vi "FGV Protokoll.vi"(6 "Enum":T1, 8 "error in (no error)":errorcluster caption="Fehler (Eingang, kein Fehler)", 9 "Graph2":waveform(dbl)[](graph), 10 "Pfad":path, 11 "Boolesch":bool) -> (0 "error out":errorcluster caption="Fehler (Ausgang)", 1 "Graph2 2":waveform(dbl)[](graph) caption="Graph2", 2 "Pfad":path, 3 "Boolesch 2":bool)   [LabVIEW 2015, in "EPA 1065.lvlib" / "Interference verificaton 1065-366.lvlib"]
uses:
  Interference verificaton 1065-366.lvlib
  Aktion FGV Protokoll.ctl
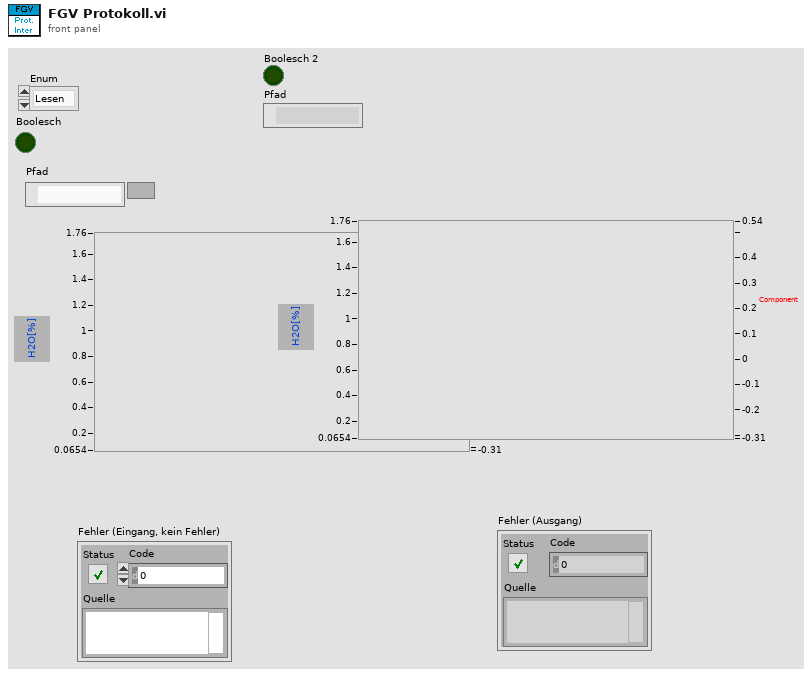
[diagram p1: front panel]
types:
  T1 = typedef "EPA 1065.lvlib/Interference verificaton 1065-366.lvlib/Aktion FGV Protokoll.ctl" = enum16{"Lesen", "ini"}
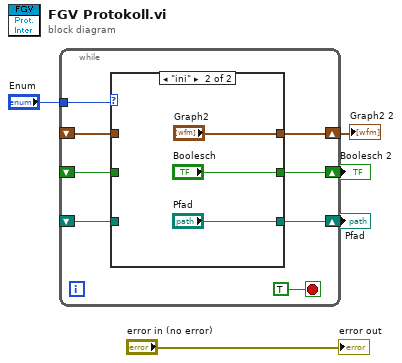
[diagram p0: block diagram]
diagram:
  n1 = while {
    tunnel: "Enum" -> [w12]
    shift-right: [w11] -> w4
    shift-left: _ -> [w9]
    shift-right: [w10] -> w3
    shift-left: _ -> [w8]
    shift-right: [w7] -> w2
    shift-left: _ -> [w6]
    stop <- TRUE stop-if-true
    n2 = case shown="\"ini\"" w12 {
      tunnel: [w16 "Boolesch"] -> w11
      tunnel: [w15 "Pfad"] -> w10
      tunnel: w9 -> [w16 _]
      tunnel: w8 -> [w15 _]
      tunnel: [w14 "Graph2"] -> w7
      tunnel: w6 -> [w14 _]
      frame "Lesen", Default {
      }
      frame "ini" {
      }
    }
  }
  "Boolesch 2" <- w4
  "Pfad" <- w3
  "Graph2 2" <- w2
  "error out" <- "error in (no error)"
